vi "Engine Simulation RT Driver VI.vi"(6 "Device Clock":string, 9 "Device Inputs FIFO":refnum<k33>, 10 "Device Outputs FIFO":refnum<k33>, 11 "Device Reference":T1 format="%.0x") -> ()   [LabVIEW 2011, in "Engine Sim RT.lvlib"]
uses:
  Engine Sim RT.lvlib
  <vilib>/NI Veristand/Custom Device API/Custom Device Item Ref.ctl
  <vilib>/Platform/TimedLoop/XDataNode/timing_clust.ctl
  <vilib>/Platform/TimedLoop/XDataNode/nitl_modes.ctl
  <vilib>/Platform/TimedLoop/XDataNode/wakeup.ctl
  <userlib>/_FPGA Interface Advanced Tools/FPGA Interface Base/FPGA Interface Base.lvclass
  <userlib>/_FPGA Interface Advanced Tools/FPGA Interface Wrapper/NiFPGA Write.vi
  <userlib>/_FPGA Interface Advanced Tools/FPGA Interface Wrapper/NiFPGA Write - U32.vi
  <userlib>/_FPGA Interface Advanced Tools/FPGA Interface Wrapper/NiFPGA Write - I32.vi
  <userlib>/_FPGA Interface Advanced Tools/FPGA Interface Wrapper/NiFPGA Write - U64.vi
  <vilib>/Utility/error.llb/Error Cluster From Error Code.vi
  <vilib>/Platform/TimedLoop/XDataNode/XDataNode.xnode
  <vilib>/Platform/TimedLoop/XDataNode/XDNodeRunTimeDep.lvlib
  <vilib>/NI Veristand/Custom Device API/Custom Device API.lvlib
  <vilib>/NI Veristand/Custom Device Tools/Custom Device Utility Library/Custom Device Utility Library.lvlib
panel:
  in  "Initialization Status Notifier":refnum<notifier>
  in  "Status Notifier":refnum<notifier>
  # "Custom Device Template\nv1.0"
  # "Use this template as a starting point for creating a custom device code module. The input controls shown here are specially named controls that the system will use to provide the device loop with data. The controls are not required for the device loop to run. For instance, if the device doesn't produce any output data, then you don't need the Device Outputs FIFO control. If you do use these controls, however, they need to have these exact names to be functional."
  # "The optional status notifier element is used to notify the RT engine of the last state of the custom device, and to indicate the device has completed execution. If this control is not used, a default No Error value is returned to the system when the device finishes execution.\n\nNote: This error state is not checked until the system shuts down. Use an output status channel to send more immediate status values to the system."
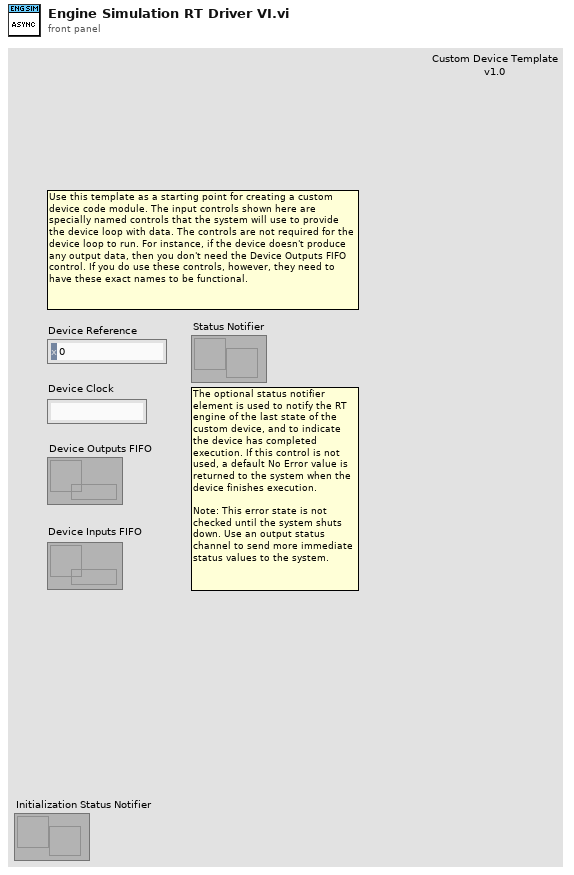
[diagram p1: front panel]
types:
  T1 = typedef "Custom Device API.lvlib/Custom Device Item Ref.ctl" = u64
  T2 = typedef "Custom Device API.lvlib/Custom Device Item Info.ctl" = cluster{"Name":string, "Is Channel":bool, "GUID":string}
  T3 = typedef "Custom Device API.lvlib/Custom Device Timed Loop Priority.ctl" = enum32{"Low", "Medium", "High"}
  T4 = typedef "Engine Sim RT.lvlib/RT Data Cluster.ctl" = cluster{"Finished Late? [i-1]":bool, "Global Start Time":i64, "Global End Time":i64, "Channel Descriptors":T5, "DevOutputs":dbl[], "DevInputs":dbl[], "OutFIFO":refnum<k33>, "InFIFO":refnum<k33>, "RAW FPGA Session":u32, "DataReplayVoltages":T12[], "Old DevInputs":dbl[]}
  T5 = typedef "Engine Simulation Shared.lvlib/Channel Descriptors.ctl" = cluster{"Write Descriptors":T6[], "Read Descriptors":T9[], "Status Descriptor":T11}
  T6 = typedef "Engine Simulation Shared.lvlib/FPGA Write Descriptor.ctl" = cluster{"Register Type":T7, "Reg Address":u32, "FIFO Idx":i32, "Reg Name":string, "Data Type":T8}
  T7 = typedef "Engine Simulation Shared.lvlib/InputChannelTypes.ctl" = enum16{"Engine Speed", "Offset"}
  T8 = typedef "niFpgaDataTypeControl.ctl" = enum32{"Boolean", "I8", "I16", "I32", "I64", "U8", "U16", "U32", "U64", "FXP", "CustomControl"}
  T9 = typedef "Engine Simulation Shared.lvlib/FPGA Read Descriptor.ctl" = cluster{"Register Type":T10, "Reg Address":u32, "FIFO Idx":i32, "DurationMultiplier":dbl, "Reg Name":string, "Data Type":T8}
  T10 = typedef "Engine Simulation Shared.lvlib/OutputChannelTypes.ctl" = enum16{"Cycle Angle", "Crank Angle", "Time Duration", "Angle Duration", "Start Angle", "End Angle"}
  T11 = typedef "Engine Simulation Shared.lvlib/Status Chan Descriptor.ctl" = cluster{"ErrorIDx":i32, "CountIDx":i32, "DurationIDx":i32}
  T12 = typedef "Engine Simulation Shared.lvlib/DataReplayVoltageConfig.ctl" = cluster{"VScaleMPath":string, "VScaleBPath":string, "DefaultVScaleM":u32, "DefaultVScaleB":i32, "EnableFIFOIdx":i32, "MFIFOIdx":i32, "BFIFOIdx":i32, "Reset":bool, "MAddress":u32, "BAddress":u32}
  T13 = typedef "XDNodeRunTimeDep.lvlib/timing_clust.ctl" = cluster{"Expected End [f-1]":u64, "Actual End [f-1]":u64, "Finished Late? [f-1]":bool, "Expected End [i-1]":u64, "Actual End [i-1]":u64, "Finished Late? [i-1]":bool, "Expected Start [i]":u64, "Actual Start [i]":u64, "Expected Start [f]":u64, "Actual Start [f]":u64, "Source Name":string, "Structure Name":string, "Period":i64, "Deadline":i64, "Offset":i64, "Start":i64, "Priority":i32, "Timeout":i32, "Mode":T14, "Wakeup Reason":T15, "Error":errorcluster, "Source Type":string, "Secondary Source Type":string, "Global End Time":u64, "Global Start Time":u64, "Frame Duration":u64, "Iteration Duration":u64, "Assigned CPU":i32, "I/O Scan Engine Mode":u32}
  T14 = typedef "XDNodeRunTimeDep.lvlib/nitl_modes.ctl" = enum32{"No Change", "Process missed periods, maintain original phase", "Discard missed periods, maintain original phase", "Process missed periods, ignore original phase", "Discard missed periods, ignore original phase"}
  T15 = typedef "XDNodeRunTimeDep.lvlib/wakeup.ctl" = enum32{"Normal", "Aborted", "Asynchronous wakeup", "Timing source error", "Timed loop error", "Timeout"}
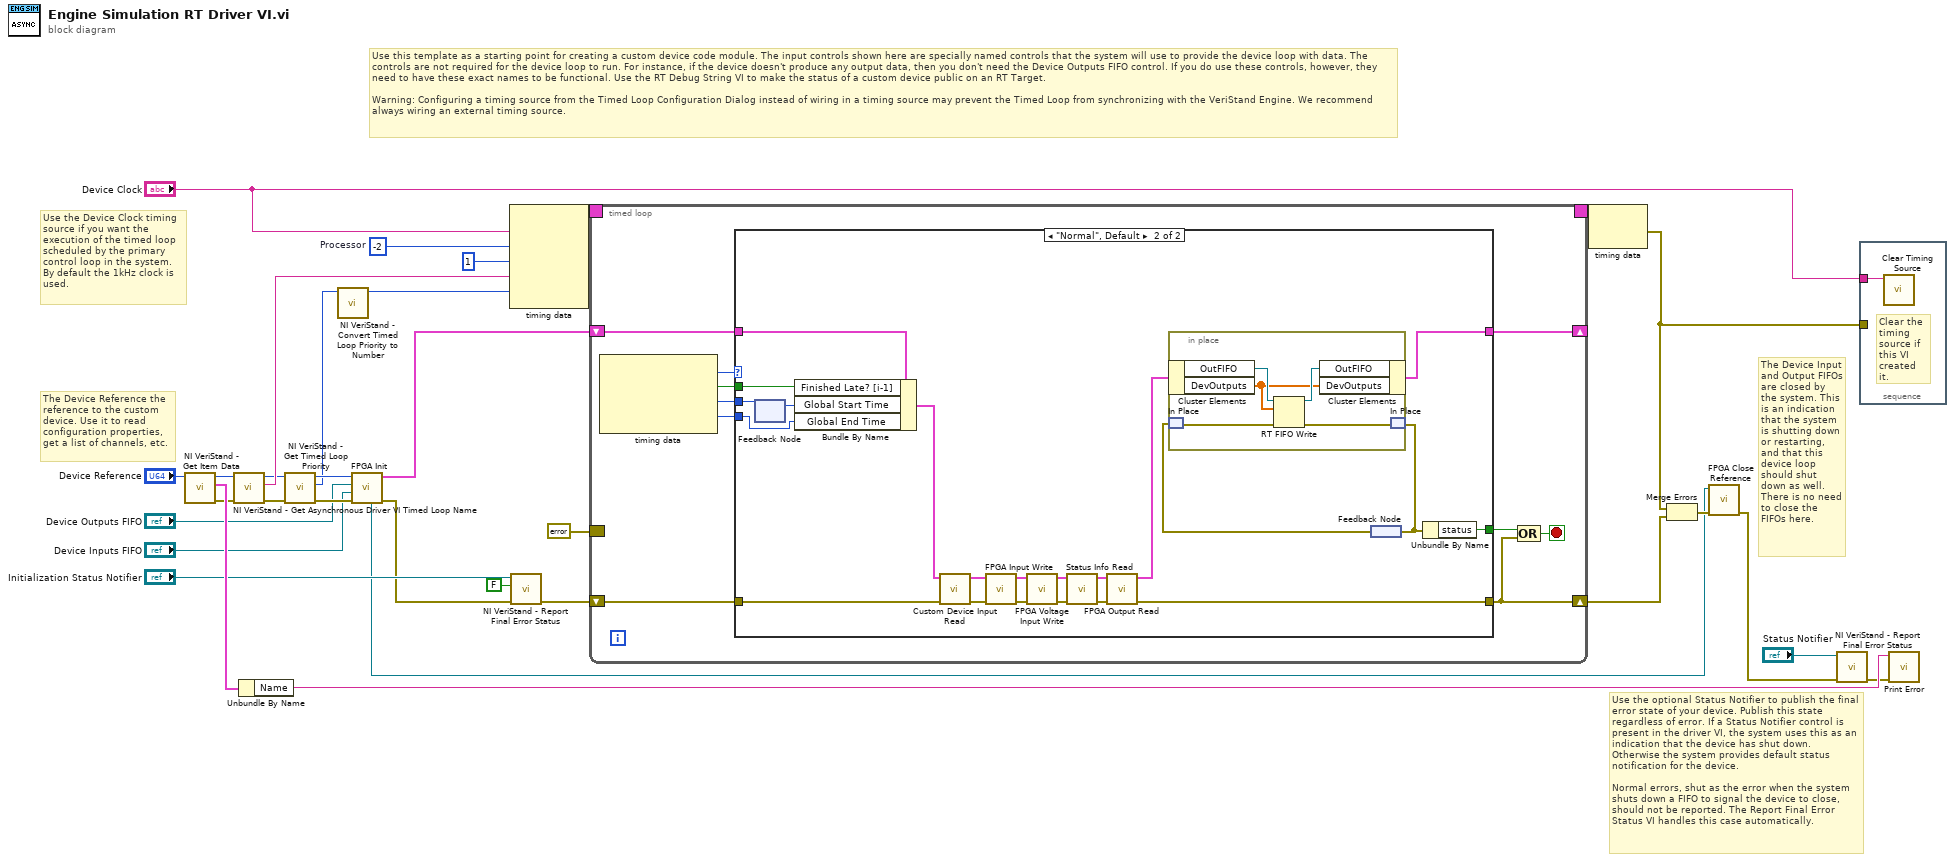
[diagram p0: block diagram]
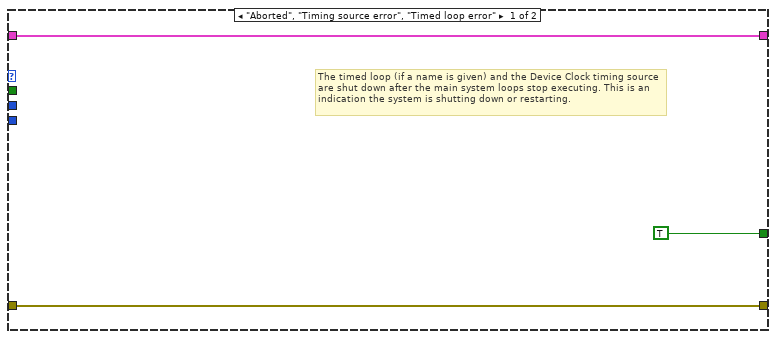
[diagram p2: hidden frame]
diagram:
  w26 = -2  # Processor
  # "Use the optional Status Notifier to publish the final error state of your device. Publish this state regardless of error. If a Status Notifier control is present in the driver VI, the system uses this as an indication that the device has shut down. Otherwise the system provides default status notification for the device.\n\nNormal errors, shut as the error when the system shuts down a FIFO to signal the device to close, should not be reported. The Report Final Error Status VI handles this case automatically."
  # "The Device Input and Output FIFOs are closed by the system. This is an indication that the system is shutting down or restarting, and that this device loop should shut down as well. There is no need to close the FIFOs here."
  # "The Device Reference the reference to the custom device. Use it to read configuration properties, get a list of channels, etc."
  # "Use the Device Clock timing source if you want the execution of the timed loop scheduled by the primary control loop in the system. \nBy default the 1kHz clock is used."
  # "Use this template as a starting point for creating a custom device code module. The input controls shown here are specially named controls that the system will use to provide the device loop with data. The controls are not required for the device loop to run. For instance, if the device doesn't produce any output data, then you don't need the Device Outputs FIFO control. If you do use these controls, however, they need to have these exact names to be functional. Use the RT Debug String VI to make the status of a custom device public on an RT Target.\n\nWarning: Configuring a timing source from the Timed Loop Configuration Dialog instead of wiring in a timing source may prevent the Timed Loop from synchronizing with the VeriStand Engine. We recommend always wiring an external timing source."
  n1 = call <vilib>:"NI VeriStand - Get Item Data.vi"("Item Ref in"="Device Reference") -> ("error out"=w10:errorcluster, "Item Info"=w18:T2, "Item Ref out"=w9:T1)  [unwired: 7 in, 1 out]
  n2 = call <vilib>:"NI VeriStand - Get Asynchronous Driver VI Timed Loop Name.vi"("error in (no error)"=w10, "Device Ref in"=w9) -> ("error out"=w8:errorcluster, "Device Timed Loop Name"=w23:string, "Device Ref out"=w7:T1)  [unwired: 7 out]
  n3 = Unbundle By Name(w18) -> ("Name"=w17:string)
  n4 = call <vilib>:"NI VeriStand - Get Timed Loop Priority.vi"("error in (no error)"=w8, "Device Ref in"=w7) -> ("error out"=w29:errorcluster, "Priority"=w28:T3, "Device Ref out"=w30:T1)  [unwired: 7 out]
  n5 = call <vilib>:"NI VeriStand - Convert Timed Loop Priority to Number.vi"("Priority"=w28) -> ("Numeric Priority"=w27:i32)  [unwired: 10 out]
  n6 = call "FPGA Init.vi"("error in (no error)"=w29, "Device Inputs FIFO"="Device Inputs FIFO", "Device Outputs FIFO"="Device Outputs FIFO", "Item Ref in"=w30) -> ("error out"=w3:errorcluster, "RT Data"=w1:T4, "FPGA Session Out"=w2:refnum<class "FPGA Interface Base.lvclass">)  [unwired: 5 in]
  n7 = node-c288("Device Clock", w26, i64 1 ("Period"), w23, w27) -> (w32:T13)
  n8 = call <vilib>:"NI VeriStand - Report Final Error Status.vi"("error in (no error)"=w3, "Filter FIFO Errors (T)"=FALSE, "Status Notifier"="Initialization Status Notifier") -> ("error out"=w12:errorcluster)  [unwired: 8 out]
  n9 = timed-loop {
    timing: w32 -> [_]
    timing-out: [_] -> w31
    shift-right: [w33] -> w22
    shift-left: w12 -> [w42]
    shift-right: [w34] -> _
    shift-left: w1 -> [w35]
    border: errorcluster {"status"=FALSE, "code"=0, "source"=""} ("error out") -> [_]
    stop <- w39 stop-if-true
    n10 = node-c288() -> (w41:T15, w38:bool, w37:i64, w36:i64)  [unwired: 1 out]
    n11 = case shown="\"Normal\", Default" w41 {
      tunnel: w42 -> [w45 w60]
      tunnel: [w45 w51] -> w33
      tunnel: [TRUE w61] -> w40
      tunnel: w38 -> [_ w66]
      tunnel: w37 -> [_ w65]
      tunnel: w36 -> [_ w64]
      tunnel: w35 -> [w43 w62]
      tunnel: [w43 w57] -> w34
      frame "Aborted", "Timing source error", "Timed loop error" {
        # "The timed loop (if a name is given) and the Device Clock timing source are shut down after the main system loops stop executing. This is an indication the system is shutting down or restarting."
      }
      frame "Normal", Default {
        n12 = feedback-in #1(w65) -> ()
        n13 = feedback #1() -> (w63:i64)  [unwired: 1 in]
        n14 = Bundle By Name(cluster=w62, "Finished Late? [i-1]"=w66, "Global Start Time"=w63, "Global End Time"=w64) -> (w47:T4)
        n15 = call "Custom Device Input Read.vi"("error in (no error)"=w60, "RT data in"=w47) -> ("error out"=w48:errorcluster, "RT data out"=w46:T4)  [unwired: 8 in]
        n16 = call "FPGA Input Write.vi"("error in (no error)"=w48, "RT data in"=w46) -> ("error out"=w53:errorcluster, "RT data out"=w52:T4)  [unwired: 8 in]
        n17 = call "FPGA Voltage Input Write.vi"("error in (no error)"=w53, "RT data in"=w52) -> ("error out"=w56:errorcluster, "RT data out"=w54:T4)  [unwired: 8 in]
        n18 = call "Status Info Read.vi"("error in (no error)"=w56, "RT data in"=w54) -> ("error out"=w55:errorcluster, "RT data out"=w50:T4)  [unwired: 8 in]
        n19 = call "FPGA Output Read.vi"("error in (no error)"=w55, "RT data in"=w50) -> ("error out"=w51:errorcluster, "RT data out"=w49:T4)  [unwired: 8 in]
        n20 = feedback #2() -> (w58:errorcluster)
        n21 = in-place {
          n22 = in-place-cluster #3(w49) -> ("OutFIFO"=w69:refnum<k33>, "DevOutputs"=w67:dbl[])
          n23 = in-place-match #4(w58) -> (w71:errorcluster)
          n24 = RT FIFO Write(0:w69, 1:w67, 3:w71) -> (8:w68:refnum<k33>, 11:w70:errorcluster)  [unwired: 2 in, 2 out]
          n25 = in-place-cluster #3("OutFIFO"=w68, "DevOutputs"=w67) -> (w57:T4)
          n26 = in-place-match #4(w70) -> (w59:errorcluster)
        }
        n27 = feedback-in #2(w59) -> ()
        n28 = Unbundle By Name(w59) -> ("status"=w61:bool)
      }
    }
    n29 = Compound Arithmetic op=OR(w40, w33) -> (w39:bool)
  }
  n30 = node-c288(w31) -> (w20:errorcluster)
  n31 = Merge Errors(w20, w22) -> (w21:errorcluster)
  n32 = call-dynamic "FPGA Close Reference.vi"("error in (no error)"=w21, "FPGA Session In"=w2) -> ("error out"=w16:errorcluster)  [unwired: 9 in]
  n33 = call <vilib>:"NI VeriStand - Report Final Error Status.vi"("error in (no error)"=w16, "Status Notifier"="Status Notifier") -> ("error out"=w15:errorcluster)  [unwired: 1 in, 8 out]
  n34 = stacked-sequence {
    tunnel: w20 -> [_]
    tunnel: "Device Clock" -> [w78]
    frame #0 {
      # "Clear the timing source if this VI created it."
      n35 = call <vilib>:"Clear Timing Source.vi"("name"=w78) -> ()  [unwired: 1 in, 10 out]
    }
  }
  n36 = call "Print Error.vi"("error in (no error)"=w15, "Your code's public name"=w17) -> ()  [unwired: 8 in, 1 out]
